vi "读取-求解.vi"(8 "error in (no error)":errorcluster caption="错误输入（无错误）", 11 "计算器类 输入":refnum<class "计算器类.lvclass">) -> (0 "error out":errorcluster caption="错误输出", 3 "计算器类 输出":refnum<class "计算器类.lvclass">)   [LabVIEW 2020, in "计算器类.lvclass"]
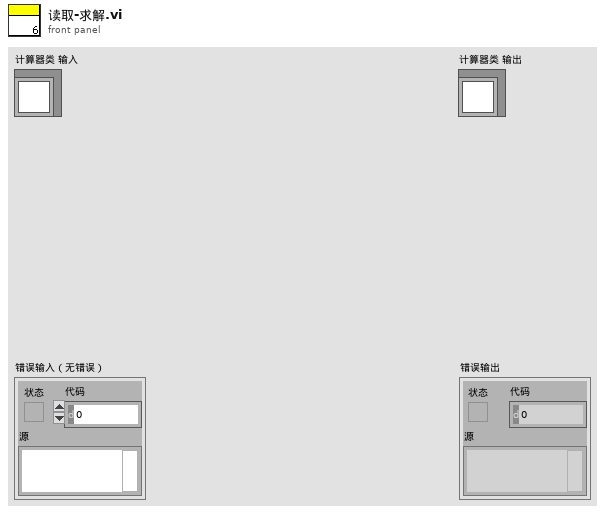
[diagram p1: front panel]
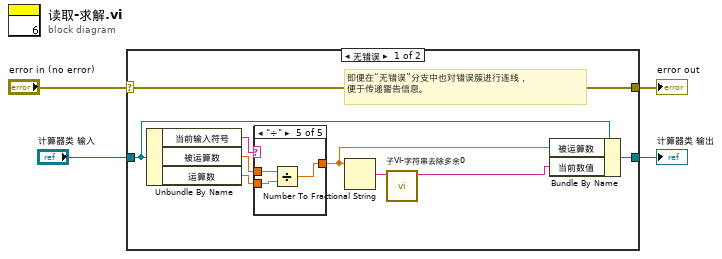
[diagram p0: block diagram]
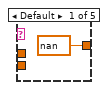
[diagram p2: hidden frame]
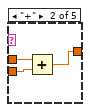
[diagram p3: hidden frame]
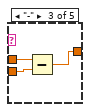
[diagram p4: hidden frame]
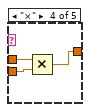
[diagram p5: hidden frame]
diagram:
  n1 = case shown="无错误" "error in (no error)" {
    selector: "error in (no error)" -> [w13 w28]
    tunnel: [w13 w28] -> w3
    tunnel: [w7 w27] -> w1
    tunnel: "计算器类 输入" -> [w8 w27]
    frame No Error {
      # "即便在“无错误”分支中也对错误簇进行连线，\n便于传递警告信息。"
      n2 = Unbundle By Name(w8) -> ("当前输入符号"=w11:string, "被运算数"=w10:dbl, "运算数"=w9:dbl)
      n3 = case shown="\"÷\"" w11 {
        tunnel: w10 -> [_ w17 w20 w23 w26]
        tunnel: [nan w16 w19 w22 w25] -> w6
        tunnel: w9 -> [_ w15 w18 w21 w24]
        frame Default {
        }
        frame "+" {
          n4 = Add(x=w17, y=w15) -> (x+y=w16:dbl)
        }
        frame "-" {
          n5 = Subtract(x=w20, y=w18) -> (x-y=w19:dbl)
        }
        frame "×" {
          n6 = Multiply(x=w23, y=w21) -> (x*y=w22:dbl)
        }
        frame "÷" {
          n7 = Divide(x=w26, y=w24) -> (x/y=w25:dbl)
        }
      }
      n8 = Number To Fractional String(number=w6) -> (F-format string=w12:string)  [unwired: 3 in]
      n9 = call "子VI-字符串去除多余0.vi"("带0字符串"=w12) -> ("result string"=w5:string)  [unwired: 10 in]
      n10 = Bundle By Name(cluster=w8, "被运算数"=w6, "当前数值"=w5) -> (w7:refnum<class "计算器类.lvclass">)
    }
    frame Error {
    }
  }
  "error out" <- w3
  "计算器类 输出" <- w1
